vi "ActionVIOnCompile.vi"(8 "error in (no error)":errorcluster, 11 "Device Item Ref in":T1 format="%.0x") -> (0 "error out":errorcluster)   [LabVIEW 2024, in "Embedded TDMS Logger System Explorer.lvlib"]
doc: "Collects the user defined System Definition of the Custom Device as defined in the System Explorer and compiles this into a transferrable format to send to the engine for execution."
uses:
  Embedded TDMS Logger System Explorer.lvlib
  <vilib>/NI VeriStand/Custom Device API/Custom Device Item Ref.ctl
  Shared/Compiled.Settings.ctl
  Shared/SegmentOptions.ctl
  Shared/File Classes/File/FileAsCluster.ctl
  Shared/File Classes/Group/GroupAsCluster.ctl
  Shared/File Classes/Channel/ChannelAsCluster.ctl
  <vilib>/NI VeriStand/Custom Device API/Data Reference.ctl
  Shared/File Classes/Meta Data.ctl
  <vilib>/NI VeriStand/Custom Device API/Get Item Property (U16).vi
  <vilib>/NI VeriStand/Custom Device API/Get Item Property (Boolean).vi
  <vilib>/NI VeriStand/Custom Device API/Get Item Property (Double).vi
  <vilib>/NI VeriStand/Custom Device API/Set Item Property (Variant).vi
  Shared/File Classes/File/File.lvclass
  <vilib>/NI VeriStand/Custom Device API/Custom Device API.lvlib
  <vilib>/NI/NIVS Inline Async API/_Data Access System Explorer/Data Access System Explorer.lvlib
  Shared/Embedded TDMS Logger Shared.lvlib
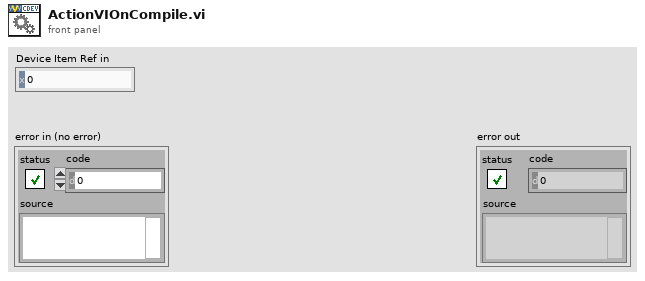
[diagram p1: front panel]
types:
  T1 = typedef "Custom Device API.lvlib/Custom Device Item Ref.ctl" = u64
  T2 = enum16{"Output/Write", "Input/Read", "Input/ReadWrite"}
  T3 = cluster{"Name":string, "Type":enum16{"Output/Write", "Input/Read", "Input/ReadWrite"}, "VS Refs":T1[]}
  T4 = typedef "Embedded TDMS Logger Shared.lvlib/Compiled.Settings.ctl" = cluster{"Name":string, "Async Init Timeout":u16, "Segment Files":bool, "Segment Every":dbl, "Segment by":T5, "dt per loop":dbl, "output cluster":T6, "Action Settings":cluster{"On Start":bool, "On Segment":bool, "On Error":bool, "Start Command":string, "Segment Command":string, "Error Command":string}}
  T5 = typedef "SegmentOptions.ctl" = enum16{"Time (s)", "Size (MB)"}
  T6 = typedef "FileAsCluster.ctl" = cluster{"Name":string, "Directory":string, "Date Captured":string, "Groups":T7[], "Meta Data":T10[], "File Start Time":timestamp, "appended path":path}
  T7 = typedef "GroupAsCluster.ctl" = cluster{"Name":string, "Channels":T8[], "Meta Data":T10[]}
  T8 = typedef "ChannelAsCluster.ctl" = cluster{"Name":string, "Data Reference":T9, "Wfm?":bool, "Decimation":i32, "Current Value":dbl, "Meta Data":T10[], "WfmPath":string}
  T9 = typedef "Custom Device API.lvlib/Data Reference.ctl" = i32
  T10 = typedef "Meta Data.ctl" = cluster{"Key":string, "Value":string}
  T11 = typedef "Custom Device API.lvlib/Custom Device Item Info.ctl" = cluster{"Name":string, "Is Channel":bool, "GUID":string, "Is Waveform":bool}
  T12 = cluster{"Name":string, "Type":enum16{"Output/Write", "Input/Read", "Input/ReadWrite"}, "VS Refs":T1[]}[]
  T13 = cluster{"On Start":bool, "On Segment":bool, "On Error":bool, "Start Command":string, "Segment Command":string, "Error Command":string}
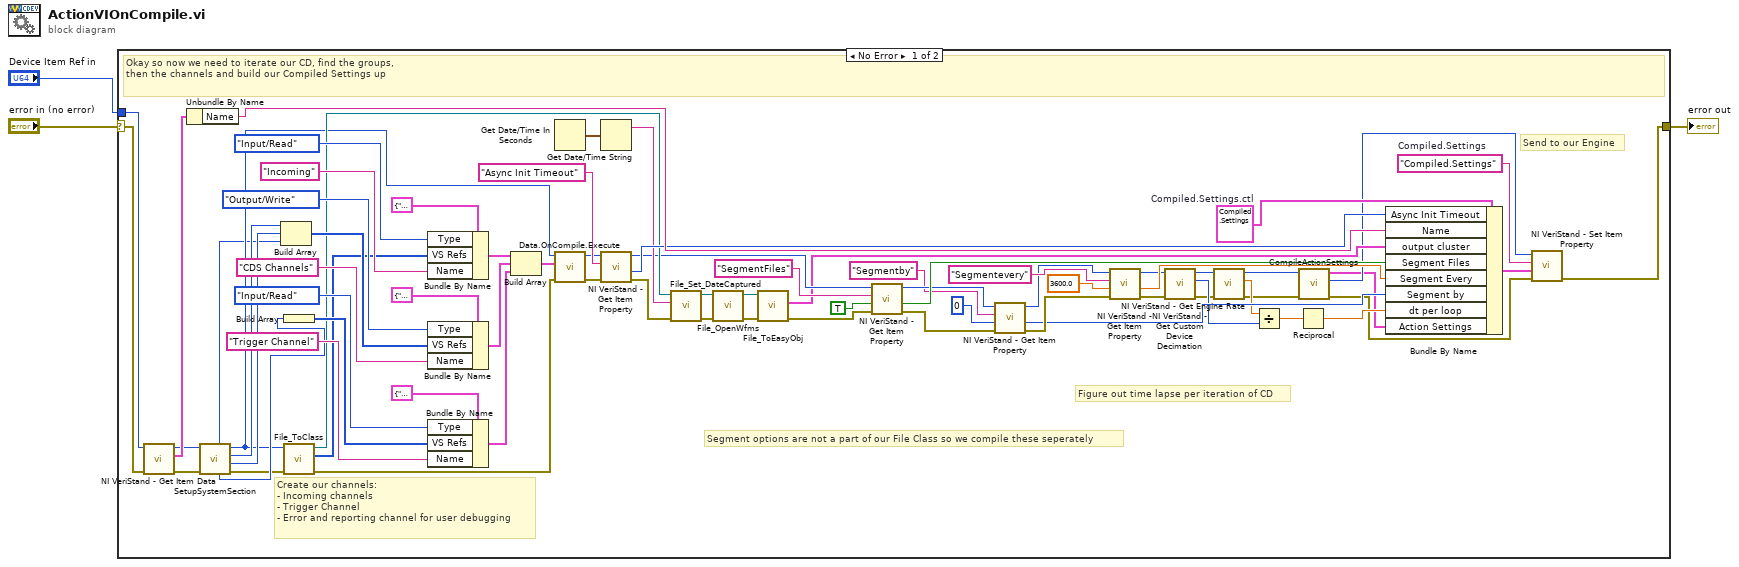
[diagram p0: block diagram]
diagram:
  n1 = case shown="No Error" "error in (no error)" {
    selector: "error in (no error)" -> [w74 w78]
    tunnel: [w75 w78] -> w3
    tunnel: "Device Item Ref in" -> [w69 _]
    frame No Error {
      w67 = T4 {"Name"="", "Async Init Timeout"=0, "Segment Files"=FALSE, "Segment Every"=0.0, "Segment by"=enum."Size (MB)", "dt per loop"=0.0, "output cluster"={"Name"="", "Directory"="", "Date Captured"="", "Groups"=[], "Meta Data"=[], "File Start Time"=timestamp(0 s since 1904-01-01), "appended path"=path ""}, "Action Settings"={"On Start"=FALSE, "On Segment"=FALSE, "On Error"=FALSE, "Start Command"="", "Segment Command"="", "Error Command"=""}}  # Compiled.Settings.ctl
      w77 = "Compiled.Settings"  # Compiled.Settings
      # "Send to our Engine"
      # "Figure out time lapse per iteration of CD"
      # "Create our channels:\n- Incoming channels\n- Trigger Channel\n- Error and reporting channel for user debugging"
      # "Segment options are not a part of our File Class so we compile these seperately"
      # "Okay so now we need to iterate our CD, find the groups,\nthen the channels and build our Compiled Settings up"
      n2 = call <vilib>:"NI VeriStand - Get Item Data.vi"("error in (no error)"=w74, "Item Ref in"=w69) -> ("error out"=w40:errorcluster, "Item Info"=w73:T11, "Item Ref out"=w41:T1)  [unwired: 6 in, 1 out]
      n3 = Unbundle By Name(w73) -> ("Name"=w72:string)
      n4 = call "SetupSystemSection.vi"("error in (no error)"=w40, "Node Ptr"=w41) -> ("error out"=w25:errorcluster, "Error Code Ref"=w26:T1, "Triggered Ref"=w27:T1, "Parent Ref Out"=w15:T1, "Trigger Ref"=w28:T1, "Logging Ref"=w9:T1)  [unwired: 4 in]
      n5 = Build Array(w27, w26, w9) -> (w39:T1[])
      n6 = Build Array(w28) -> (w30:T1[])
      n7 = call "File_ToClass.vi"("error in (no error)"=w25, "Item Ref in"=w15) -> ("error out"=w17:errorcluster, "Channels"=w24:T1[], "File out"=w23:refnum<class "File.lvclass">)  [unwired: 7 in]
      n8 = Bundle By Name(cluster=T3 {"Name"="", "Type"=enum."Output/Write", "VS Refs"=[]} ("Group"), "Type"=T2."Input/Read", "VS Refs"=w24, "Name"="Incoming" ("Item Name")) -> (w34:T3)
      n9 = Bundle By Name(cluster=T3 {"Name"="", "Type"=enum."Output/Write", "VS Refs"=[]} ("Group"), "Type"=T2."Output/Write", "VS Refs"=w39, "Name"="CDS Channels") -> (w35:T3)
      n10 = Bundle By Name(cluster=T3 {"Name"="", "Type"=enum."Output/Write", "VS Refs"=[]} ("Group"), "Type"=T2."Input/Read", "VS Refs"=w30, "Name"="Trigger Channel") -> (w29:T3)
      n11 = Build Array(w34, w35, w29) -> (w50:T12)
      n12 = Get Date/Time In Seconds() -> (seconds since 1Jan1904=w68:timestamp)
      n13 = call <vilib>:"Data.OnCompile.Execute.vi"("error in"=w17, "VS Ref Groups"=w50, "Custom Device Ref"=w15) -> ("error out"=w16:errorcluster, "Custom Device Ref"=w14:T1)  [unwired: 7 in]
      n14 = Get Date/Time String(seconds (now)=w68) -> (date string=w22:string)  [unwired: 2 in, 1 out]
      n15 = call-poly <vilib>:"NI VeriStand - Get Item Property.vi"("error in (no error)"=w16, "Property Name"="Async Init Timeout", "Item Ref in"=w14) -> ("error out"=w18:errorcluster, "Value"=w70:u16, "Item Ref out"=w21:T1)  [unwired: 5 in, 1 out]
      n16 = call-dynamic "File_Set_DateCaptured.vi"("error in (no error)"=w18, "Date Captured"=w22, "File in"=w23) -> ("error out"=w10:errorcluster, "File out"=w13:refnum<class "File.lvclass">)  [unwired: 7 in]
      n17 = call-dynamic "File_OpenWfms.vi"("error in (no error)"=w10, "File in"=w13) -> ("error out"=w11:errorcluster, "File out"=w12:refnum<class "File.lvclass">)  [unwired: 8 in]
      n18 = call-dynamic "File_ToEasyObj.vi"("error in (no error)"=w11, "File in"=w12) -> ("error out"=w19:errorcluster, "output cluster"=w20:T6)  [unwired: 7 in, 1 out]
      n19 = call-poly <vilib>:"NI VeriStand - Get Item Property.vi"("error in (no error)"=w19, "Default Value"=TRUE, "Property Name"="SegmentFiles", "Item Ref in"=w21) -> ("error out"=w63:errorcluster, "Value"=w64:bool, "Item Ref out"=w62:T1)  [unwired: 4 in, 1 out]
      n20 = call-poly <vilib>:"NI VeriStand - Get Item Property.vi"("error in (no error)"=w63, "Default Value"=u16 0, "Property Name"="Segmentby", "Item Ref in"=w62) -> ("error out"=w57:errorcluster, "Value"=w54:u16, "Item Ref out"=w56:T1)  [unwired: 4 in, 1 out]
      n21 = call-poly <vilib>:"NI VeriStand - Get Item Property.vi"("error in (no error)"=w57, "Default Value"=3600.0, "Property Name"="Segmentevery", "Item Ref in"=w56) -> ("error out"=w43:errorcluster, "Value"=w55:dbl, "Item Ref out"=w42:T1)  [unwired: 4 in, 1 out]
      n22 = call <vilib>:"NI VeriStand - Get Custom Device Decimation.vi"("error in (no error)"=w43, "Device Ref in"=w42) -> ("error out"=w44:errorcluster, "Decimation"=w48:i32, "Device Ref out"=w45:T1)  [unwired: 7 in]
      n23 = call <vilib>:"NI VeriStand - Get Engine Rate.vi"("error in (no error)"=w44, "Item Ref in"=w45) -> ("error out"=w5:errorcluster, "Rate (Hz)"=w49:dbl, "Item Ref out"=w6:T1)  [unwired: 7 in]
      n24 = Divide(x=w49, y=w48) -> (x/y=w47:dbl)
      n25 = Reciprocal(x=w47) -> (1/x=w46:dbl)
      n26 = call "CompileActionSettings.vi"("error in (no error)"=w5, "Item Ref in"=w6) -> ("error out"=w4:errorcluster, "Item Ref out"=w8:T1, "Action Settings"=w7:T13)  [unwired: 7 in]
      n27 = Bundle By Name(cluster=w67, "Async Init Timeout"=w70, "Name"=w72, "output cluster"=w20, "Segment Files"=w64, "Segment Every"=w55, "Segment by"=w54, "dt per loop"=w46, "Action Settings"=w7) -> (w76:T4)
      n28 = call-poly <vilib>:"NI VeriStand - Set Item Property.vi"("error in (no error)"=w4, "Value"=w76, "Property Name"=w77, "Item Ref in"=w8) -> ("error out"=w75:errorcluster)  [unwired: 5 in, 2 out]
    }
    frame Error {
    }
  }
  "error out" <- w3
